vi "Main.vi"() -> ()   [LabVIEW 2013]
doc: "Main code that will run on the robot and contains all the logic and hardware interfaces."
uses:
  cRIO_Code/Data/TypeDefs/UTM Location.ctl
  cRIO_Code/Data/TypeDefs/Sail Set Suggestions.ctl
  cRIO_Code/Data/TypeDefs/Rudder Set Suggestions.ctl
  cRIO_Code/Data/TypeDefs/OverrideInformation.ctl
  cRIO_Code/Data/TypeDefs/OverrideMode.ctl
  cRIO_Code/Logic/Classes/Missions/GenericMission/GenericMission.lvclass
  cRIO_Code/Logic/Classes/Obstacle/Obstacle.lvclass
  cRIO_Code/Data/TypeDefs/BoatType.ctl
  cRIO_Code/Logic/Classes/Logger/Logger.lvclass
panel:
  in  "Calibration VI Path":path=path "cRIO_Code/Logic/Hindbrain/Hardware_Interfaces/Simple RC to Dynamixel/RC_calibration.vi"
  in  "Boat Type":T1=enum."Damn Yankee"
  in  "Do Basic Logging? (T)":bool
  out "Logging file path":path
  out "Missions":refnum<class "GenericMission.lvclass">[](array[class])
  out "Obstacles":refnum<class "Obstacle.lvclass">[](array[class])
  out "Finished Missions":refnum<class "GenericMission.lvclass">[](array[class])
  out "OverrideInformation":T2={"OverrideMode"=enum."Rudder", "SailSetting"={"MainSailSuggestion"=0.0, "JibSailSuggestion"=0.0}, "Rudder Setpoint"=0.0, "Sim_Wind_Speed"=0.0, "Sim_Wind_Heading"=0.0} {"SailSetting"."MainSailSuggestion" min=0.0 max=1.0; "SailSetting"."JibSailSuggestion" min=0.0 max=1.0; "Rudder Setpoint" min=-0.95 max=0.95 scale=1.0..-1.0}
  out "DisplayCounter":i32
  out "AbsWindDirection":dbl
  out "IronsRange":dbl
  out "RudderPosition":T5 min=-0.95 max=0.95 scale=1.0..-1.0
  out "SailPositions":T4 {"MainSailSuggestion" min=0.0 max=1.0; "JibSailSuggestion" min=0.0 max=1.0}
  out "RelWindDirection":dbl
  out "RateOfTurn":dbl
  out "BoatLocation":T6 {"North" format="%#_10f"; "East" format="%#_8f"}
  out "BoatDirection":dbl
  out "WindSpeed":dbl
  out "BoatSpeed":dbl
  in  "XBee Serial Port":refnum<visa-resource-name>="COM8"
  in  "stop":bool
  # "ALL THE DEBUG INFO - Eric"
  # "SET THIS BEFORE RUNNING\nOR YOU WILL NEED TO\nRESTART THE CODE!!!"
  # "For Little Boat Initialization"
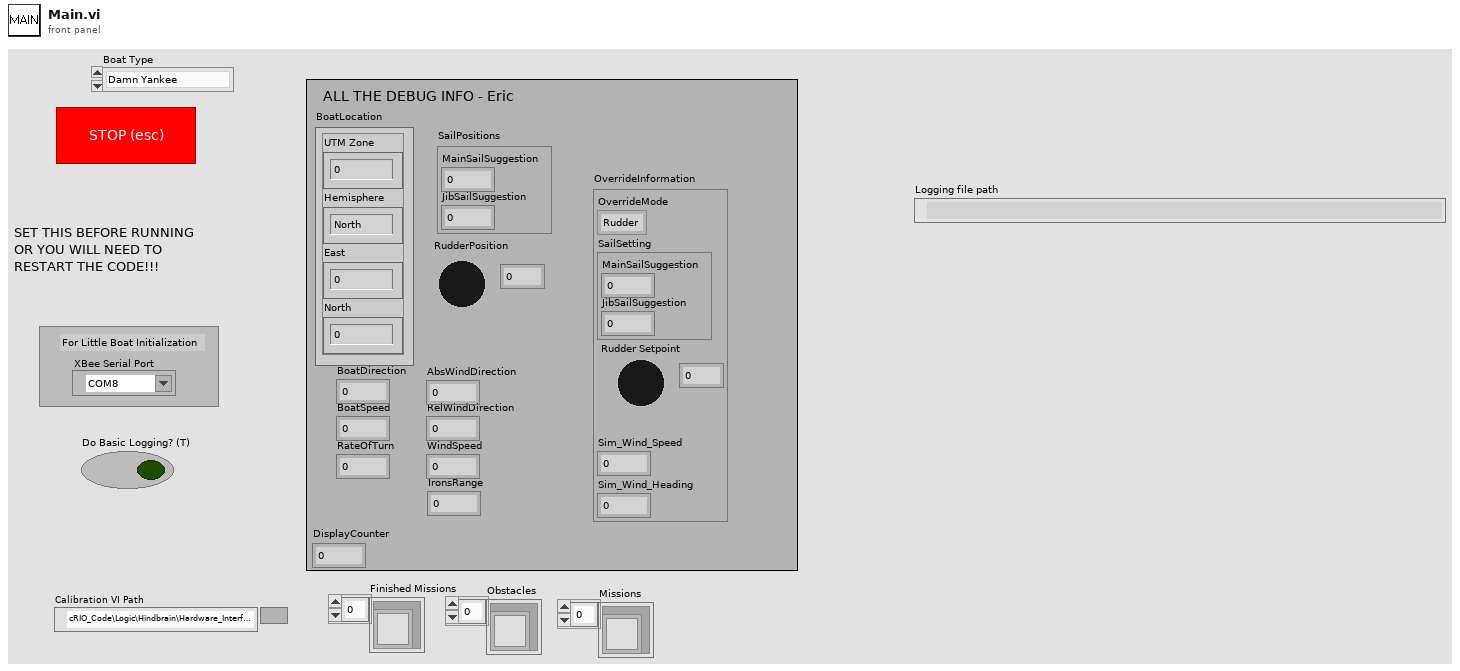
[diagram p1: front panel]
types:
  T1 = typedef "BoatType.ctl" = enum16{"Blackbody Radiation", "ReadLog", "Little boats", "Simulation", "Damn Yankee"}
  T2 = typedef "OverrideInformation.ctl" = cluster{"OverrideMode":T3, "SailSetting":T4, "Rudder Setpoint":T5, "Sim_Wind_Speed":dbl, "Sim_Wind_Heading":dbl}
  T3 = typedef "OverrideMode.ctl" = enum16{"None", "Rudder", "Sails", "Both"}
  T4 = typedef "Sail Set Suggestions.ctl" = cluster{"MainSailSuggestion":dbl, "JibSailSuggestion":dbl}
  T5 = typedef "Rudder Set Suggestions.ctl" = dbl
  T6 = typedef "UTM Location.ctl" = cluster{"UTM Zone":dbl, "Hemisphere":enum16{"North", "South"}, "East":dbl, "North":dbl}
  T7 = enum32{"Invalid", "Standard", "Closed", "Hidden", "Minimized", "Maximized"}
  T8 = typedef "MissionNotifiers.ctl" = cluster{"Missions":refnum<notifier>, "Finished Missions":refnum<notifier>, "Obstacles":refnum<notifier>}
  T9 = typedef "Notifiers.ctl" = cluster{"BoatSpeed":refnum<notifier>, "WindSpeed":refnum<notifier>, "EStop":refnum<notifier>, "BoatDirection":refnum<notifier>, "Luffing":refnum<notifier>, "RudderForce":refnum<notifier>, "BatteryVoltage":refnum<notifier>, "StayForces":refnum<notifier>, "BoatLocation":refnum<notifier>, "Pitch":refnum<notifier>, "Roll":refnum<notifier>, "RateOfTurn":refnum<notifier>, "RelWindDirection":refnum<notifier>, "SailPositions":refnum<notifier>, "RudderPosition":refnum<notifier>, "IronsRange":refnum<notifier>, "AbsWindDirection":refnum<notifier>, "OverrideInformation":refnum<notifier>, "DynamixelTorques":refnum<notifier>, "MotorSetup":refnum<notifier>, "AirmarStatus":refnum<notifier>, "HardwareOnline?":refnum<notifier>, "Sim_ActualSailPositions [0,1]":refnum<notifier>, "DynamixelCycleTracker":refnum<notifier>, "BoatVelocityDirection":refnum<notifier>, "SimWindHeading(rad)":refnum<notifier>, "SimWindSpeed(m/s)":refnum<notifier>, "RCInputValues":refnum<notifier>, "Finished Waypoints":refnum<notifier>, "DesiredHeading":refnum<notifier>, "Latest Mission ID":refnum<notifier>, "Latest Obstacle ID":refnum<notifier>, "DownwindDiscouragedRange":refnum<notifier>, "Tack Range":refnum<notifier>, "Tacking?":refnum<notifier>}
  T10 = typedef "Queues.ctl" = cluster{"Waypoints":refnum<queue>}
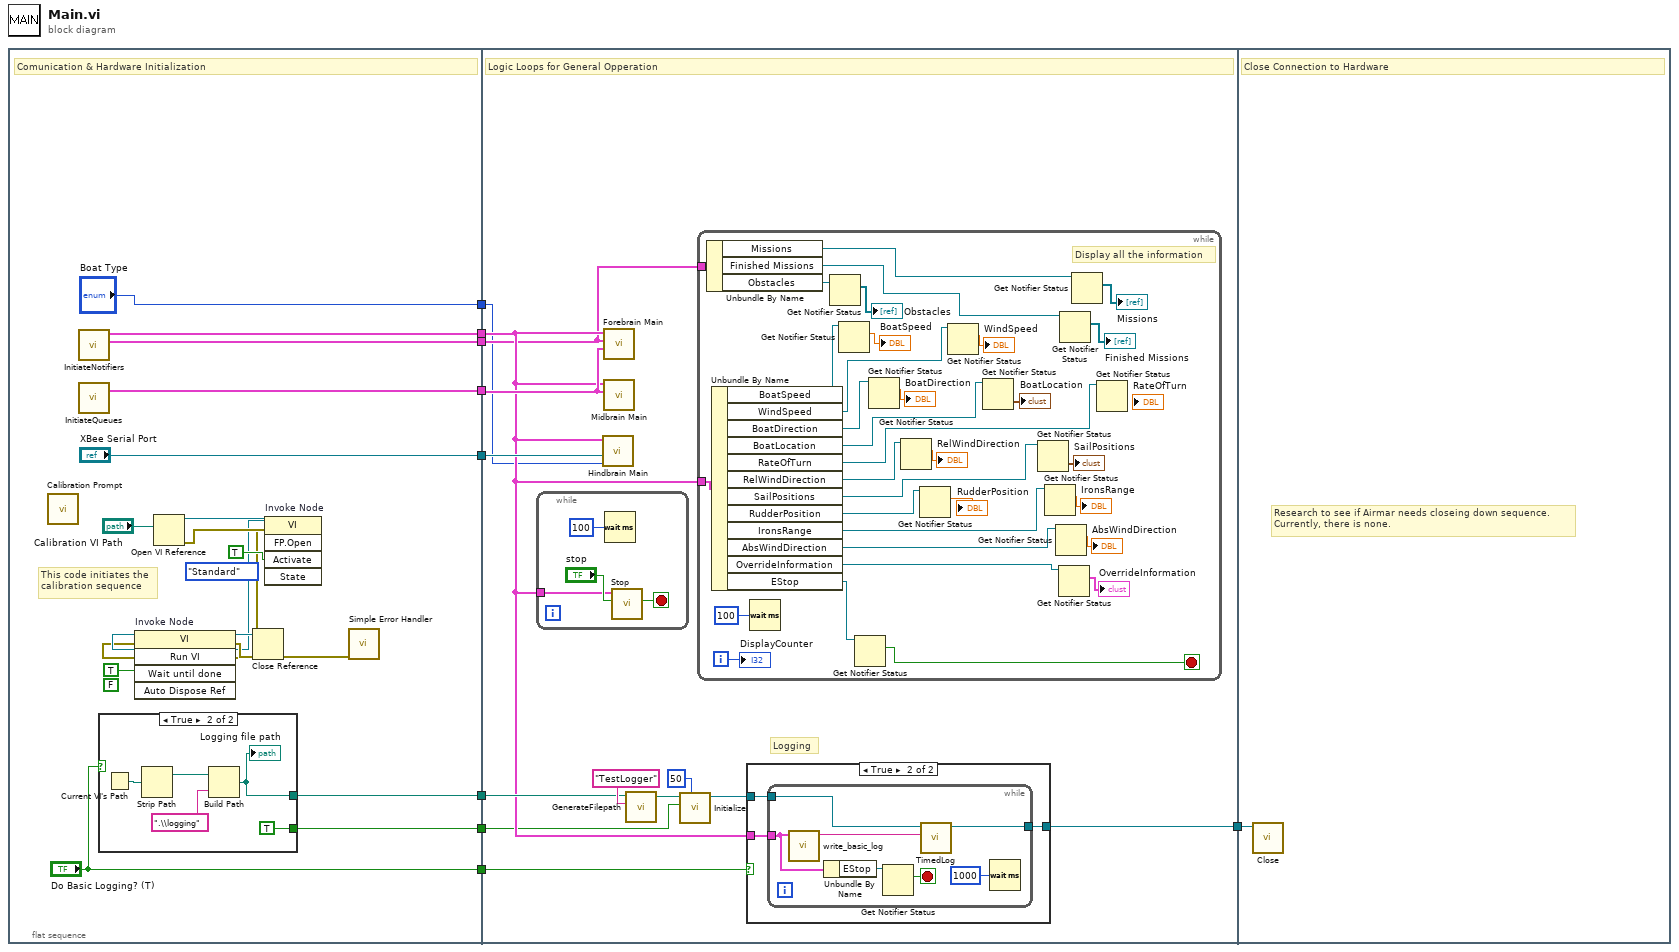
[diagram p0: block diagram]
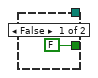
[diagram p2: hidden frame]
diagram:
  n1 = flat-sequence {
    tunnel: [w27] -> w9
    tunnel: ["Boat Type"] -> w8
    tunnel: [w26] -> w7
    tunnel: ["XBee Serial Port"] -> w6
    tunnel: [w24] -> w5
    tunnel: [w23] -> w3
    tunnel: [w22] -> w2
    tunnel: ["Do Basic Logging? (T)"] -> w1
    tunnel: w9 -> [w45]
    tunnel: w8 -> [w34]
    tunnel: w7 -> [w38]
    tunnel: w6 -> [w46]
    tunnel: w5 -> [w37]
    tunnel: [w41] -> w4
    tunnel: w3 -> [w39]
    tunnel: w2 -> [w36]
    tunnel: w1 -> [w35]
    tunnel: w4 -> [w95]
    frame #0 {
      (unwired) FALSE ("Auto Dispose Reference")
      (unwired) T7."Standard" ("State")
      # "This code initiates the\ncalibration sequence"
      # "Comunication & Hardware Initialization"
      n2 = call "Calibration Prompt"() -> ()  [unwired: 10 in, 2 out]
      n3 = call "InitiateNotifiers.vi"() -> ("Mission Notifiers"=w24:T8, "NotifierReferences"=w26:T9)  [unwired: 9 in, 1 out]
      n4 = call "InitiateQueues.vi"() -> ("Queue References"=w27:T10)  [unwired: 3 in]
      n5 = case shown="True" "Do Basic Logging? (T)" {
        tunnel: [_ w32] -> w23
        tunnel: [FALSE ("Enable? (T)") TRUE ("Enable? (T)")] -> w22
        frame False {
        }
        frame True {
          n6 = Current VI's Path() -> (path=w30:path)
          n7 = Strip Path(path=w30) -> (stripped path=w29:path)  [unwired: 1 out]
          n8 = Build Path(base path=w29, name or relative path=".\\logging") -> (appended path=w32:path)
          "Logging file path" <- w32
        }
      }
      n9 = Open VI Reference(vi path="Calibration VI Path") -> (vi reference=w18:refnum<vi>, error out=w17:errorcluster)  [unwired: 1 in, 4 out]
      n10 = invoke on="Invoke Node" class="VI" method="FP.Open"(reference=w18, error in=w17, "Activate"=TRUE ("Activate?")) -> (reference out=w11:refnum<vi>, error out=w10:errorcluster)  [unwired: 2 in, 3 out]
      n11 = invoke on="Invoke Node" class="VI" method="Run VI"(reference=w11, error in=w10, "Wait until done"=TRUE ("Wait Until Done")) -> (reference out=w13:refnum<vi>, error out=w12:errorcluster)  [unwired: 2 in, 3 out]
      n12 = Close Reference(reference=w13, error in (no error)=w12) -> (error out=w16:errorcluster)
      n13 = call <vilib>:"Simple Error Handler.vi"("error in (no error)"=w16) -> ()  [unwired: 1 in, 8 out]
    }
    frame #1 {
      # "Logging"
      # "Logic Loops for General Opperation"
      n14 = while {
        tunnel: w38 -> [w91]
        stop <- w92 stop-if-true
        n15 = Wait (ms)(milliseconds to wait=u32 100) -> ()  [unwired: 1 out]
        n16 = call "Stop.vi"("StopButton"="stop", "NotifierReff"=w91) -> ("StopOut"=w92:bool)  [unwired: 9 in]
      }
      n17 = call "Hindbrain Main.vi"("Boat Type"=w34, "XBee Serial Port"=w46, "NotifierReff"=w38) -> ()  [unwired: 9 in]
      n18 = call "Forebrain Main.vi"("QueueRef"=w45, "Mission Notifiers"=w37, "NotifierReff"=w38) -> ()  [unwired: 8 in, 1 out]
      n19 = call "Midbrain Main.vi"("Waypoint Queue Ref"=w45, "Notifier Ref"=w38) -> ()  [unwired: 10 in]
      n20 = call "GenerateFilepath.vi"("Identifier"="TestLogger", "Data storage folder"=w39) -> ("File path out"=w42:path)  [unwired: 8 in, 1 out]
      n21 = call "Initialize.vi"("buffer size"=50, "Enable? (T)"=w36, "File path"=w42) -> ("Logger out"=w43:refnum<class "Logger.lvclass">)  [unwired: 7 in, 1 out]
      n22 = while {
        tunnel: w38 -> [w89]
        tunnel: w37 -> [w64]
        i -> [w69]
        stop <- w66 stop-if-true
        # "Display all the information"
        n23 = Unbundle By Name(w64) -> ("Missions"=w59:refnum<notifier>, "Finished Missions"=w61:refnum<notifier>, "Obstacles"=w63:refnum<notifier>)
        n24 = Unbundle By Name(w89) -> ("BoatSpeed"=w88:refnum<notifier>, "WindSpeed"=w86:refnum<notifier>, "BoatDirection"=w83:refnum<notifier>, "BoatLocation"=w82:refnum<notifier>, "RateOfTurn"=w80:refnum<notifier>, "RelWindDirection"=w78:refnum<notifier>, "SailPositions"=w77:refnum<notifier>, "RudderPosition"=w75:refnum<notifier>, "IronsRange"=w72:refnum<notifier>, "AbsWindDirection"=w70:refnum<notifier>, "OverrideInformation"=w68:refnum<notifier>, "EStop"=w65:refnum<notifier>)
        n25 = Wait (ms)(milliseconds to wait=u32 100) -> ()  [unwired: 1 out]
        n26 = Get Notifier Status(notifier=w63) -> (current notification=→"Obstacles":refnum<class "Obstacle.lvclass">[])  [unwired: 1 in, 4 out]
        n27 = Get Notifier Status(notifier=w88) -> (current notification=→"BoatSpeed":dbl)  [unwired: 1 in, 4 out]
        n28 = Get Notifier Status(notifier=w65) -> (current notification=w66:bool)  [unwired: 1 in, 4 out]
        n29 = Get Notifier Status(notifier=w83) -> (current notification=→"BoatDirection":dbl)  [unwired: 1 in, 4 out]
        n30 = Get Notifier Status(notifier=w78) -> (current notification=→"RelWindDirection":dbl)  [unwired: 1 in, 4 out]
        n31 = Get Notifier Status(notifier=w75) -> (current notification=→"RudderPosition":T5)  [unwired: 1 in, 4 out]
        n32 = Get Notifier Status(notifier=w86) -> (current notification=→"WindSpeed":dbl)  [unwired: 1 in, 4 out]
        n33 = Get Notifier Status(notifier=w82) -> (current notification=→"BoatLocation":T6)  [unwired: 1 in, 4 out]
        n34 = Get Notifier Status(notifier=w77) -> (current notification=→"SailPositions":T4)  [unwired: 1 in, 4 out]
        n35 = Get Notifier Status(notifier=w72) -> (current notification=→"IronsRange":dbl)  [unwired: 1 in, 4 out]
        n36 = Get Notifier Status(notifier=w70) -> (current notification=→"AbsWindDirection":dbl)  [unwired: 1 in, 4 out]
        n37 = Get Notifier Status(notifier=w68) -> (current notification=→"OverrideInformation":T2)  [unwired: 1 in, 4 out]
        n38 = Get Notifier Status(notifier=w61) -> (current notification=→"Finished Missions":refnum<class "GenericMission.lvclass">[])  [unwired: 1 in, 4 out]
        n39 = Get Notifier Status(notifier=w59) -> (current notification=→"Missions":refnum<class "GenericMission.lvclass">[])  [unwired: 1 in, 4 out]
        n40 = Get Notifier Status(notifier=w80) -> ()  [unwired: 1 in, 5 out]
        "DisplayCounter" <- w69
      }
      n41 = case shown="True" w35 {
        tunnel: w43 -> [w47 w50]
        tunnel: [w47 w49] -> w41
        tunnel: w38 -> [_ w48]
        frame False {
        }
        frame True {
          n42 = while {
            tunnel: w48 -> [w52]
            tunnel: w50 -> [w54]
            tunnel: [w53] -> w49
            stop <- w56 stop-if-true
            n43 = call "write_basic_log.vi"("NotifierReff"=w52) -> ("xml string"=w51:string)  [unwired: 10 in]
            n44 = Unbundle By Name(w52) -> ("EStop"=w57:refnum<notifier>)
            n45 = Get Notifier Status(notifier=w57) -> (current notification=w56:bool)  [unwired: 1 in, 4 out]
            n46 = call "TimedLog.vi"("Message"=w51, "Logger in"=w54) -> ("Logger out"=w53:refnum<class "Logger.lvclass">)  [unwired: 7 in, 2 out]
            n47 = Wait (ms)(milliseconds to wait=u32 1000) -> ()  [unwired: 1 out]
          }
        }
      }
    }
    frame #2 {
      # "Research to see if Airmar needs closeing down sequence.\nCurrently, there is none."
      # "Close Connection to Hardware"
      n48 = call "Close.vi"("Logger in"=w95) -> ()  [unwired: 10 in, 1 out]
    }
  }
